vi "ArrayView.vi"() -> ()   [LabVIEW 2011]
uses:
  <vilib>/Heliosphere Research LLC/Advanced Plotting Toolkit/Advanced Plotting Toolkit.lvlib
  <vilib>/Heliosphere Research LLC/Advanced Plotting Toolkit/properties/Colormap_Map.ctl
  <vilib>/Heliosphere Research LLC/Advanced Plotting Toolkit/properties/Colormap_Scaling.ctl
  <vilib>/Heliosphere Research LLC/Advanced Plotting Toolkit/properties/Colormap.ctl
  <vilib>/Heliosphere Research LLC/Advanced Plotting Toolkit/properties/Display.ctl
  <vilib>/Heliosphere Research LLC/Advanced Plotting Toolkit/api_plotting/ArrayViewProperties.ctl
  <vilib>/Heliosphere Research LLC/Advanced Plotting Toolkit/api_plotting/ArrayViewBoundaries.ctl
panel:
  in  "Colormap.Map":T1=enum."White-Blue"
  in  "Boundaries":T2={"X Min"=nan, "X Max"=nan, "Y Min"=nan, "Y Max"=nan}
  out "Color Plot":picture
  # "ArrayView"
  # "This example demonstrates the simplest way to visualize a\n2D array: by plotting it in pseudocolor.\n\nEach point is assigned a color, depending on the desired\ncolormap.  Then, the array is displayed as a smooth,\ncontinuous colored surface.  Try changing the colormap.\n\nBy default, the edges of the colored surface range from 0\nto NX-1 and NY-1, where NX and NY are the number of\nelements along each array dimension.  Try changing this\nbelow using the Boundaries cluster."
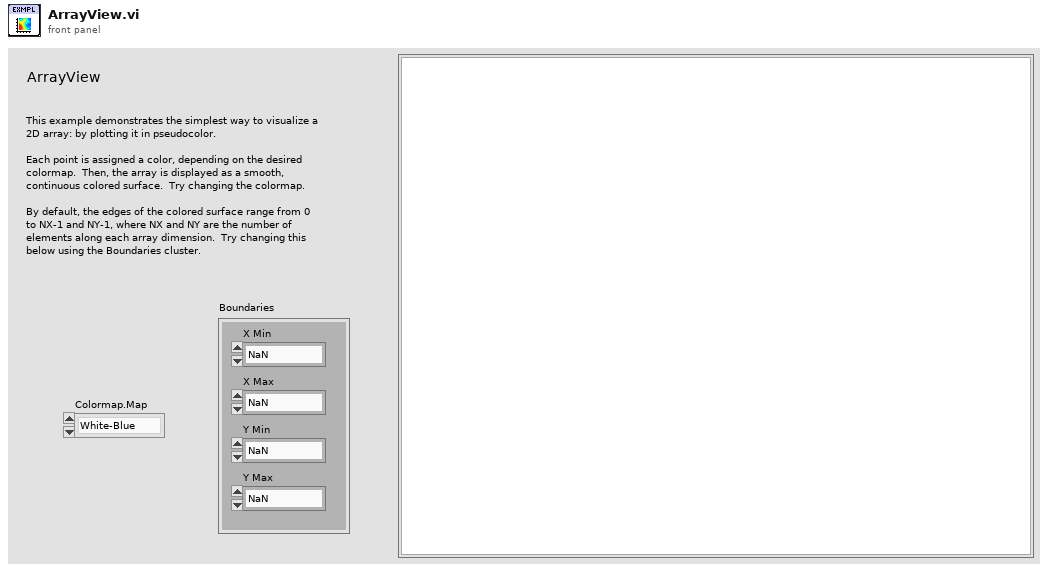
[diagram p1: front panel]
types:
  T1 = typedef "Advanced Plotting Toolkit.lvlib/Colormap_Map.ctl" = enum16{"Automatic", "Rainbow", "Hot and Cold", "White-Black", "White-Blue", "White-Green", "White-Red", "Fire", "Water", "Earth", "Air", "Pastel", "Banded", "Stepped"}
  T2 = typedef "Advanced Plotting Toolkit.lvlib/ArrayViewBoundaries.ctl" = cluster{"X Min":dbl, "X Max":dbl, "Y Min":dbl, "Y Max":dbl}
  T3 = typedef "Advanced Plotting Toolkit.lvlib/ArrayViewProperties.ctl" = cluster{"Colormap":T4, "Display":T6}
  T4 = typedef "Advanced Plotting Toolkit.lvlib/Colormap.ctl" = cluster{"Map":T1, "Value Min":dbl, "Value Max":dbl, "Scaling":T5, "Reverse":bool}
  T5 = typedef "Advanced Plotting Toolkit.lvlib/Colormap_Scaling.ctl" = enum16{"Default"}
  T6 = typedef "Advanced Plotting Toolkit.lvlib/Display.ctl" = cluster{"Alpha":dbl, "Z Order":dbl}
  T7 = typedef "Advanced Plotting Toolkit.lvlib/PlotID.ctl" = i32
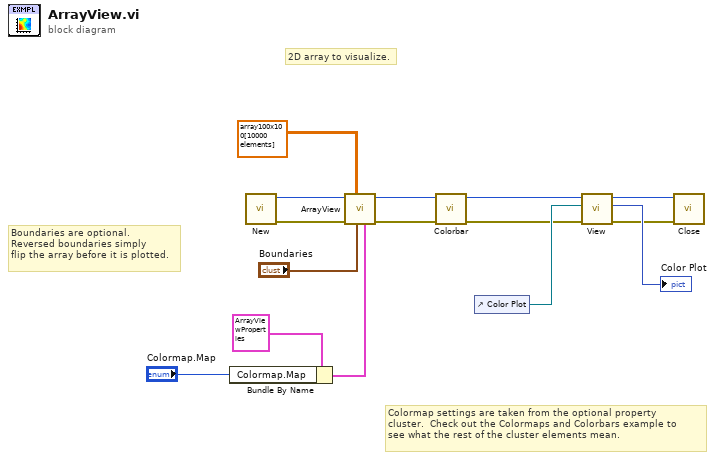
[diagram p0: block diagram]
diagram:
  # "Colormap settings are taken from the optional property\ncluster.  Check out the Colormaps and Colorbars example to\nsee what the rest of the cluster elements mean."
  # "Boundaries are optional.\nReversed boundaries simply\nflip the array before it is plotted."
  # "2D array to visualize."
  n1 = Bundle By Name(cluster=T3 {"Colormap"={"Map"=enum."Automatic", "Value Min"=nan, "Value Max"=nan, "Scaling"=enum."Default", "Reverse"=FALSE}, "Display"={"Alpha"=nan, "Z Order"=nan}} ("Array View Properties"), "Colormap.Map"="Colormap.Map") -> (w3:T3)
  n2 = call <vilib>:"New.vi"() -> ("error out"=w11:errorcluster, "Plot ID"=w12:T7)  [unwired: 10 in]
  n3 = call <vilib>:"ArrayView.vi"("Properties"=w3, "Boundaries"="Boundaries", "Data"=dbl[][] array100x100[10000 elements] ("x/y"), "error in (no error)"=w11, "Plot ID"=w12) -> ("error out"=w9:errorcluster, "Plot ID Out"=w10:T7)  [unwired: 5 in]
  n4 = call <vilib>:"Colorbar.vi"("error in (no error)"=w9, "Plot ID"=w10) -> ("error out"=w7:errorcluster, "Plot ID Out"=w8:T7)  [unwired: 8 in]
  n5 = control-ref of="Color Plot"() -> (w15:refnum<vi>)
  n6 = call <vilib>:"View.vi"("error in (no error)"=w7, "Ref for Sizing"=w15, "Plot ID"=w8) -> ("error out"=w1:errorcluster, "Picture"=→"Color Plot":picture, "Plot ID Out"=w13:T7)  [unwired: 6 in]
  n7 = call <vilib>:"Close.vi"("error in (no error)"=w1, "Plot ID"=w13) -> ()  [unwired: 9 in, 1 out]
